vi "FGV.CheckIfVIRegistered.vi"(9 "VI Ref in":refnum<vi>, 10 "VI Status":T1[](array[typedef])) -> (1 "Index of VI Ref":i32, 2 "VI Registered":bool)   [LabVIEW 2017, in "JKI Simple Localization.lvlib"]
uses:
  API/JKI Simple Localization.lvlib
  Definitions/Private/VI Info.ctl
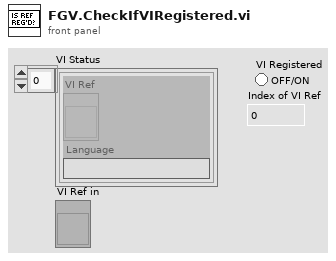
[diagram p1: front panel]
types:
  T1 = typedef "JKI Simple Localization.lvlib/VI Info.ctl" = cluster{"VI Ref":refnum<vi>, "Language":string}
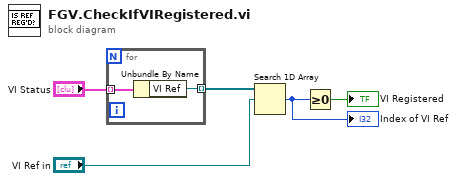
[diagram p0: block diagram]
diagram:
  n1 = for {
    tunnel: "VI Status" -> [w7] mode=indexing
    tunnel: [w6] -> w5 mode=indexing
    n2 = Unbundle By Name(w7) -> ("VI Ref"=w6:refnum<vi>)
  }
  n3 = Search 1D Array(1D array=w5, element="VI Ref in") -> (index of element=w2:i32)  [unwired: 1 in]
  "Index of VI Ref" <- w2
  n4 = Greater Or Equal To 0?(x=w2) -> (x >= 0?=→"VI Registered":bool)
